vi "devicelist-insert-info.vi"(8 "info":T3, 9 "name":string, 11 "device-list":T2(array[cluster])) -> (3 "device-list output":T2(array[cluster]))   [LabVIEW 2019]
panel:
  out "device 2":T1
  in  "device":T1
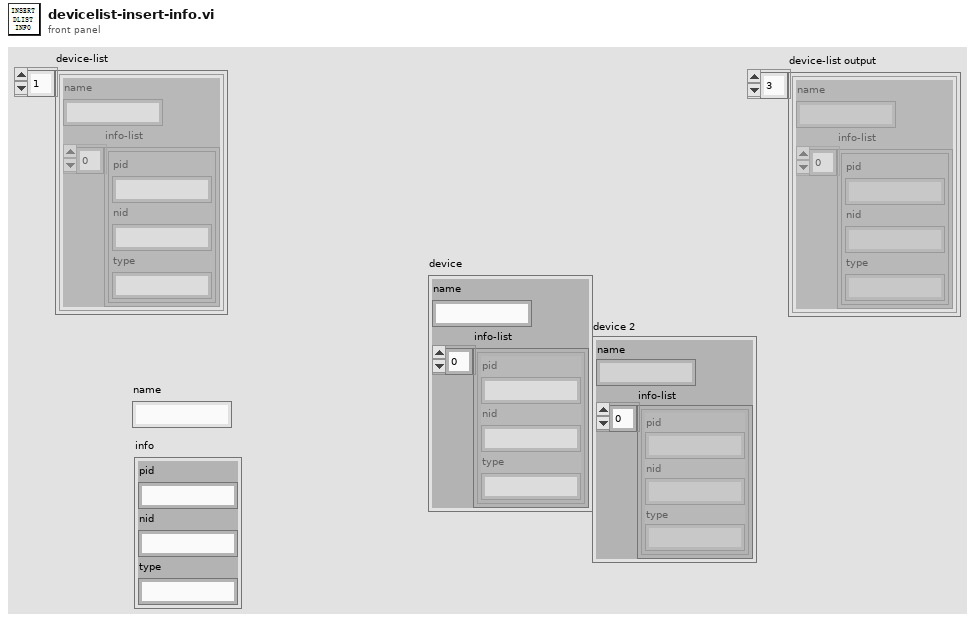
[diagram p1: front panel]
types:
  T1 = cluster{"name":string, "info-list":cluster{"pid":string, "nid":string, "type":string}[]}
  T2 = cluster{"name":string, "info-list":cluster{"pid":string, "nid":string, "type":string}[]}[]
  T3 = cluster{"pid":string, "nid":string, "type":string}
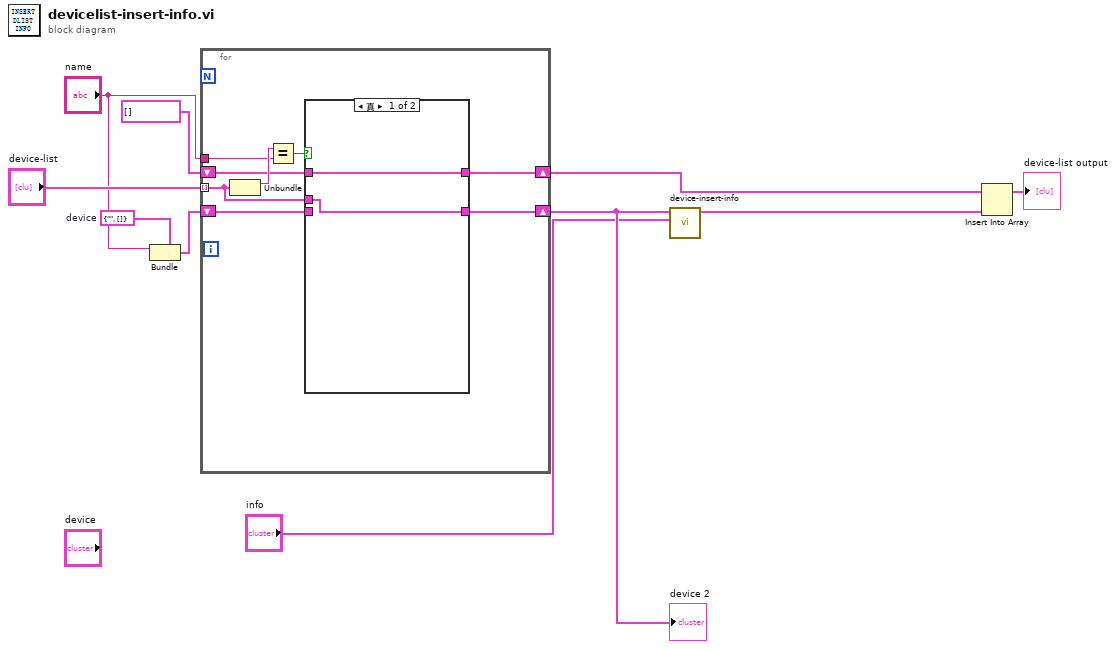
[diagram p0: block diagram]
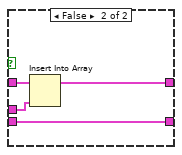
[diagram p2: hidden frame]
diagram:
  w8 = T1 {"name"="", "info-list"=[]}  # device
  n1 = Bundle(cluster=w8, "name"="name") -> (w7:T1)  [unwired: 1 in]
  n2 = for {
    tunnel: "device-list" -> [w15] mode=indexing
    tunnel: "name" -> [w17]
    shift-right: [w14] -> w3
    shift-left: T2 [] -> [w13]
    shift-right: [w12] -> w5
    shift-left: w7 -> [w11]
    n3 = Unbundle(w15) -> ("name"=w18:string)  [unwired: 1 out]
    n4 = Equal?(x=w18, y=w17) -> (x = y?=w16:bool)
    n5 = case shown="真" w16 {
      tunnel: w15 -> [w19 w22]
      tunnel: [w20 w24] -> w14
      tunnel: w13 -> [w20 w23]
      tunnel: [w19 w21] -> w12
      tunnel: w11 -> [_ w21]
      frame True {
      }
      frame False {
        n6 = Insert Into Array(array=w23, new element=w22) -> (w24:T2)  [unwired: 1 in]
      }
    }
  }
  "device 2" <- w5
  n7 = call "device-insert-info.vi"("info"="info", "device"=w5) -> ("device output"=w2:T1)  [unwired: 9 in]
  n8 = Insert Into Array(array=w3, new element=w2) -> (→"device-list output":T2)  [unwired: 1 in]
